vi "prep.vi"(8 "error in (no error)":errorcluster, 9 "Coordinate System":enum16{"Cartesian", "Cylindrical", "Spherical"}(ring), 10 "Plot processed data In":T1 caption="Data In", 11 "Line in":refnum<class "Line.lvclass">) -> (0 "error out":errorcluster, 2 "Plot processed Data Out":T1 caption="Data Out", 3 "Line out":refnum<class "Line.lvclass">)   [LabVIEW 2017, in "Line.lvclass"]
uses:
  <vilib>/Native 3D Graph/classes/Line/Line.lvclass
  <vilib>/Native 3D Graph/xcontrol/Processed Data.ctl
  <vilib>/Native 3D Graph/typedefs/plot_rep_array.ctl
  <vilib>/Native 3D Graph/typedefs/plot_rep.ctl
  <vilib>/Native 3D Graph/typedefs/range_cluster.ctl
  <vilib>/Native 3D Graph/typedefs/min_max.ctl
  <vilib>/Native 3D Graph/typedefs/plot_rep_mesh_data.ctl
  <vilib>/Native 3D Graph/classes/Line/Line.lvclass/Line.ctl
  <vilib>/Analysis/coordinate.llb/3D Coordinate Conversion (Scalar).vi
  <vilib>/Native 3D Graph/classes/Base Datatype.lvclass
  <vilib>/Native 3D Graph/xcontrol/3DPC_SurfacePlot.xctl
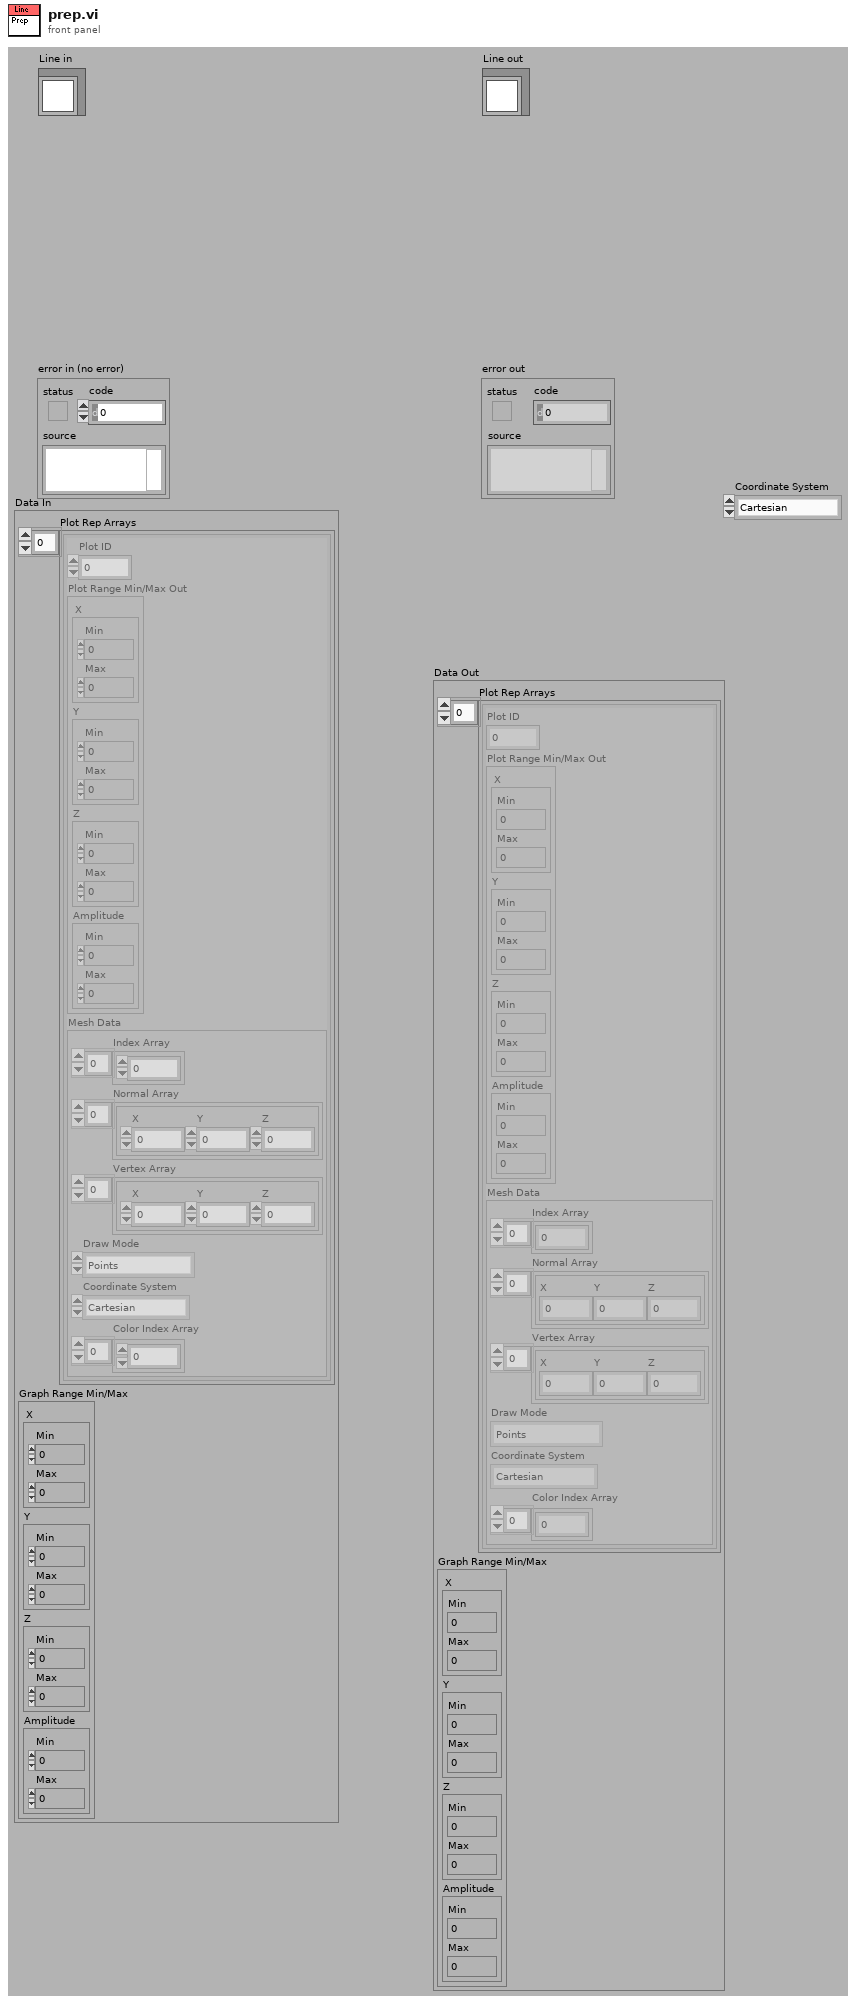
[diagram p1: front panel]
types:
  T1 = typedef "Processed Data.ctl" = cluster{"Plot Rep Arrays":T2, "Graph Range Min/Max":T4}
  T2 = typedef "3DPC_SurfacePlot.xctl/plot_rep_array.ctl" = T3[]
  T3 = typedef "3DPC_SurfacePlot.xctl/plot_rep.ctl" = cluster{"Plot ID":i32, "Plot Range Min/Max Out":T4, "Mesh Data":T6}
  T4 = typedef "3DPC_SurfacePlot.xctl/range_cluster.ctl" = cluster{"X":T5, "Y":T5, "Z":T5, "Amplitude":T5}
  T5 = typedef "3DPC_SurfacePlot.xctl/min_max.ctl" = cluster{"Min":sgl, "Max":sgl}
  T6 = typedef "3DPC_SurfacePlot.xctl/plot_rep_mesh_data.ctl" = cluster{"Index Array":u32[], "Normal Array":cluster{"X":sgl, "Y":sgl, "Z":sgl}[], "Vertex Array":cluster{"X":sgl, "Y":sgl, "Z":sgl}[], "Draw Mode":enum16{"Points", "Lines", "Line Strip", "Line Loop", "Triangles", "Triangle Strip", "Triangle Fan", "Quads", "Quad Strip", "Polygon"}, "Coordinate System":enum16{"Cartesian", "Cylindrical", "Spherical"}, "Color Index Array":i32[]}
  T7 = enum16{"Points", "Lines", "Line Strip", "Line Loop", "Triangles", "Triangle Strip", "Triangle Fan", "Quads", "Quad Strip", "Polygon"}
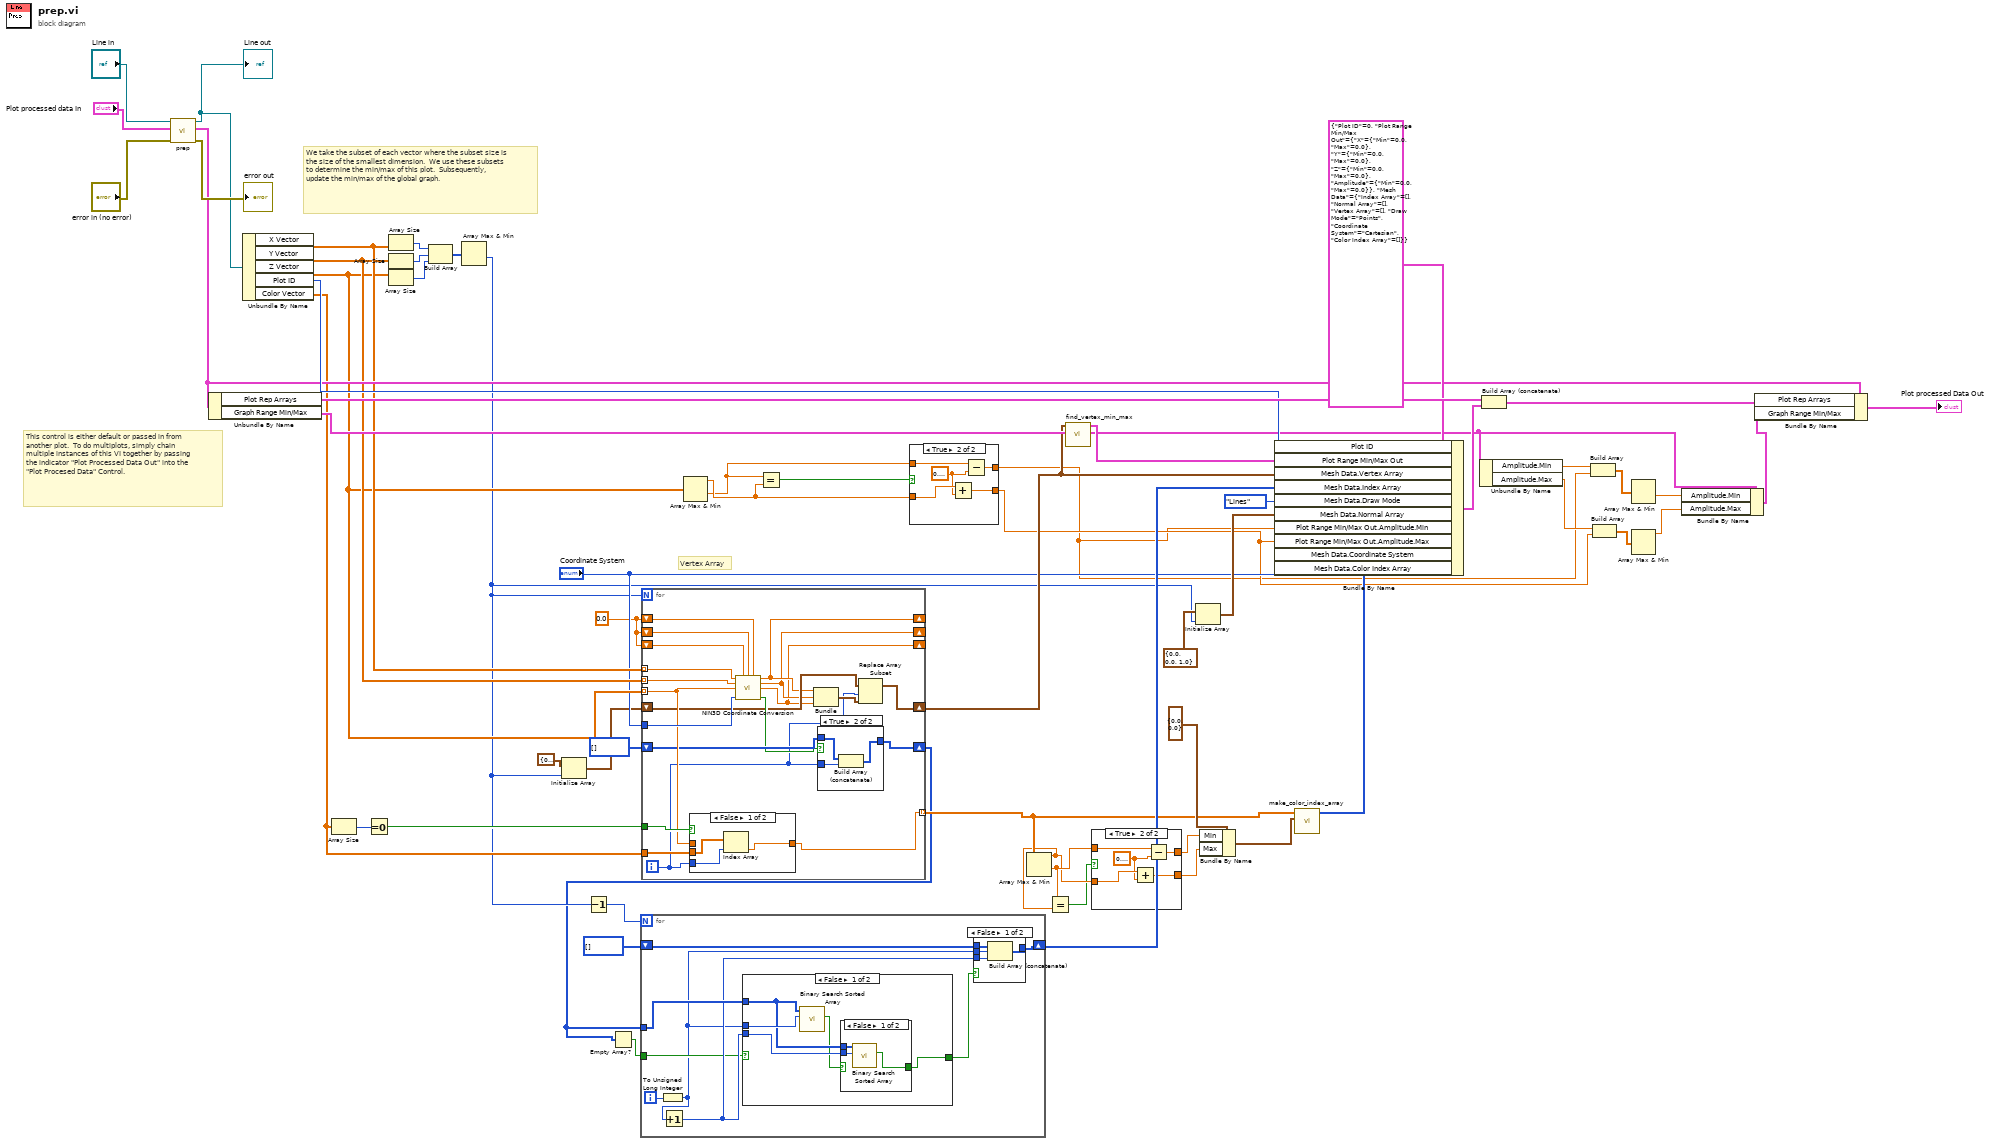
[diagram p0: block diagram]
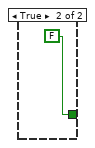
[diagram p6: hidden frame]
diagram:
  w3 = sgl 0.0
  # "We take the subset of each vector where the subset size is the size of the smallest dimension.  We use these subsets to determine the min/max of this plot.  Subsequently, update the min/max of the global graph."
  # "This control is either default or passed in from another plot.  To do multiplots, simply chain multiple instances of this VI together by passing the indicator \"Plot Processed Data Out\" into the \"Plot Procesed Data\" Control."
  # "Vertex Array"
  n1 = call-parent "prep.vi"("error in (no error)"="error in (no error)", "Plot processed data In"="Plot processed data In", "Base Datatype in"="Line in") -> ("error out"=→"error out":errorcluster, "Plot processed Data Out"=w41:T1, "Base Datatype out"=w57:refnum<class "Line.lvclass">)  [unwired: 1 in, 5 out]
  "Line out" <- w57
  n2 = Unbundle By Name(w41) -> ("Plot Rep Arrays"=w56:T2, "Graph Range Min/Max"=w39:T4)
  n3 = Unbundle By Name(w57) -> ("X Vector"=w37:sgl[], "Y Vector"=w36:sgl[], "Z Vector"=w34:sgl[], "Plot ID"=w42:i32, "Color Vector"=w20:sgl[])
  n4 = Array Size(array=w20) -> (size(s)=w24:i32)
  n5 = Equal To 0?(x=w24) -> (x = 0?=w23:bool)
  n6 = Array Size(array=w37) -> (size(s)=w53:i32)
  n7 = Array Size(array=w36) -> (size(s)=w52:i32)
  n8 = Array Size(array=w34) -> (size(s)=w51:i32)
  n9 = Build Array(w53, w52, w51) -> (w50:i32[])
  n10 = Array Max & Min(array=w50) -> (min value=w6:i32)  [unwired: 3 out]
  n11 = Initialize Array(cluster{"X":sgl, "Y":sgl, "Z":sgl} {"X"=0.0, "Y"=0.0, "Z"=0.0} ("3D Point"), w6) -> (w4:cluster{"X":sgl, "Y":sgl, "Z":sgl}[])
  n12 = Decrement(x=w6) -> (x-1=w43:i32)
  n13 = for {
    N: w6 -> [_]
    shift-right: [w70] -> w35
    shift-left: w4 -> [w71]
    tunnel: w37 -> [w81] mode=indexing
    tunnel: w36 -> [w80] mode=indexing
    tunnel: w34 -> [w77] mode=indexing
    tunnel: "Coordinate System" -> [w79]
    tunnel: w23 -> [w78]
    tunnel: [w75] -> w13 mode=indexing
    tunnel: w20 -> [w76]
    shift-right: [w72] -> w2
    shift-left: u32[] [] -> [w74]
    shift-right: [w64] -> _
    shift-left: w3 -> [w67]
    shift-right: [w63] -> _
    shift-left: w3 -> [w66]
    shift-right: [w62] -> _
    shift-left: w3 -> [w65]
    i -> [w68]
    n14 = case shown="False" w78 {
      tunnel: w77 -> [_ w89]
      tunnel: [w86 w89] -> w75
      tunnel: w76 -> [w87 _]
      tunnel: w68 -> [w88 _]
      frame False {
        n15 = Index Array(array=w87, index=w88) -> (element=w86:sgl)
      }
      frame True {
      }
    }
    n16 = call <vilib>:"NIN3D Coordinate Conversion.vi"("X"=w81, "Z_prev"=w65, "Y_prev"=w66, "X_prev"=w67, "Y"=w80, "Z"=w77, "Coordinate System"=w79) -> ("X out"=w64:sgl, "Y out"=w63:sgl, "Z out"=w62:sgl, "NaN?"=w73:bool)  [unwired: 5 in]
    n17 = Bundle("X out"=w64, "Y out"=w63, "Z out"=w62) -> (w69:cluster{"X out":sgl, "Y out":sgl, "Z out":sgl})  [unwired: 1 out]
    n18 = case shown="True" w73 {
      tunnel: w74 -> [w82 w85]
      tunnel: [w82 w84] -> w72
      tunnel: w68 -> [_ w83]
      frame False {
      }
      frame True {
        n19 = Build Array (concatenate)(w85, w83) -> (w84:u32[])
      }
    }
    n20 = Replace Array Subset(array=w71, new element=w69, index=w68) -> (w70:cluster{"X":sgl, "Y":sgl, "Z":sgl}[])
  }
  n21 = Empty Array?(array=w2) -> (empty?=w1:bool)
  n22 = for {
    N: w43 -> [_]
    shift-right: [w96] -> w47
    shift-left: u32[] [] ("Indices") -> [w97]
    tunnel: w2 -> [w94]
    tunnel: w1 -> [w92]
    i -> [w91]
    n23 = To Unsigned Long Integer(number=w91) -> (unsigned 32bit integer=w90:u32)
    n24 = Increment(x=w90) -> (x+1=w93:u32)
    n25 = case shown="False" w92 {
      tunnel: [w103 FALSE] -> w95
      tunnel: w94 -> [w105 _]
      tunnel: w90 -> [w107 _]
      tunnel: w93 -> [w106 _]
      frame False {
        n26 = call <vilib>:"Binary Search Sorted Array.vi"("Element"=w107, "Sorted Array"=w105) -> ("Found?"=w104:bool)  [unwired: 9 in]
        n27 = case shown="False" w104 {
          selector: w104 -> [_ w111]
          tunnel: w106 -> [w110 _]
          tunnel: w105 -> [w109 _]
          tunnel: [w108 w111] -> w103
          frame False {
            n28 = call <vilib>:"Binary Search Sorted Array.vi"("Element"=w110, "Sorted Array"=w109) -> ("Found?"=w108:bool)  [unwired: 9 in]
          }
          frame True {
          }
        }
      }
      frame True {
      }
    }
    n29 = case shown="False" w95 {
      tunnel: w97 -> [w101 w102]
      tunnel: [w100 w102] -> w96
      tunnel: w93 -> [w99 _]
      tunnel: w90 -> [w98 _]
      frame False {
        n30 = Build Array (concatenate)(w101, w98, w99) -> (w100:u32[])
      }
      frame True {
      }
    }
  }
  n31 = Array Max & Min(array=w34) -> (max value=w15:sgl, min value=w14:sgl)  [unwired: 2 out]
  n32 = Equal?(x=w14, y=w15) -> (x = y?=w18:bool)
  n33 = case shown="True" w18 {
    tunnel: w15 -> [w114 w119]
    tunnel: [w114 w118] -> w17
    tunnel: w14 -> [w113 w117]
    tunnel: [w113 w116] -> w16
    frame False {
    }
    frame True {
      w115 = sgl 0.1 ("y")
      n34 = Add(x=w119, y=w115) -> (x+y=w118:sgl)
      n35 = Subtract(x=w117, y=w115) -> (x-y=w116:sgl)
    }
  }
  n36 = Array Max & Min(array=w13) -> (max value=w9:sgl, min value=w10:sgl)  [unwired: 2 out]
  n37 = Equal?(x=w10, y=w9) -> (x = y?=w8:bool)
  n38 = call <vilib>:"find_vertex_min_max.vi"("Total Range Min/Max"=w39, "Vertex Array"=w35) -> ("Total Range Out"=w26:T4, "This Range Min/Max Out"=w38:T4)  [unwired: 8 out]
  n39 = case shown="True" w8 {
    tunnel: w9 -> [w121 w126]
    tunnel: [w121 w125] -> w11
    tunnel: w10 -> [w120 w124]
    tunnel: [w120 w123] -> w12
    frame False {
    }
    frame True {
      w122 = sgl 0.1 ("y")
      n40 = Add(x=w126, y=w122) -> (x+y=w125:sgl)
      n41 = Subtract(x=w124, y=w122) -> (x-y=w123:sgl)
    }
  }
  n42 = Initialize Array(cluster{"X":sgl, "Y":sgl, "Z":sgl} {"X"=0.0, "Y"=0.0, "Z"=1.0} ("3D Point"), w6) -> (w44:cluster{"X":sgl, "Y":sgl, "Z":sgl}[])
  n43 = Bundle By Name(cluster=T5 {"Min"=0.0, "Max"=0.0} ("Amplitude"), "Min"=w12, "Max"=w11) -> (w21:T5)
  n44 = call <vilib>:"make_color_index_array.vi"("Amplitude Min/Max"=w21, "Z array"=w13) -> ("Color Index Array"=w19:i32[])  [unwired: 9 out]
  n45 = Bundle By Name(cluster=T3 {"Plot ID"=0, "Plot Range Min/Max Out"={"X"={"Min"=0.0, "Max"=0.0}, "Y"={"Min"=0.0, "Max"=0.0}, "Z"={"Min"=0.0, "Max"=0.0}, "Amplitude"={"Min"=0.0, "Max"=0.0}}, "Mesh Data"={"Index Array"=[], "Normal Array"=[], "Vertex Array"=[], "Draw Mode"=enum."Points", "Coordinate System"=enum."Cartesian", "Color Index Array"=[]}} ("Plot Representation"), "Plot ID"=w42, "Plot Range Min/Max Out"=w38, "Mesh Data.Vertex Array"=w35, "Mesh Data.Index Array"=w47, "Mesh Data.Draw Mode"=T7."Lines", "Mesh Data.Normal Array"=w44, "Plot Range Min/Max Out.Amplitude.Min"=w16, "Plot Range Min/Max Out.Amplitude.Max"=w17, "Mesh Data.Coordinate System"="Coordinate System", "Mesh Data.Color Index Array"=w19) -> (w55:T3)
  n46 = Unbundle By Name(w26) -> ("Amplitude.Min"=w32:sgl, "Amplitude.Max"=w29:sgl)
  n47 = Build Array (concatenate)(w56, w55) -> (w54:T2)
  n48 = Build Array(w32, w16) -> (w31:sgl[])
  n49 = Build Array(w29, w17) -> (w28:sgl[])
  n50 = Array Max & Min(array=w31) -> (min value=w30:sgl)  [unwired: 3 out]
  n51 = Array Max & Min(array=w28) -> (max value=w27:sgl)  [unwired: 3 out]
  n52 = Bundle By Name(cluster=w26, "Amplitude.Min"=w30, "Amplitude.Max"=w27) -> (w25:T4)
  n53 = Bundle By Name(cluster=w41, "Plot Rep Arrays"=w54, "Graph Range Min/Max"=w25) -> (→"Plot processed Data Out":T1)
